vi "ToggleOnPress.vi"(11 "Input":bool) -> (3 "Output":bool)   [LabVIEW 2016]
doc: "Output becomes true Time Limit ms after Input becomes true and stays true"
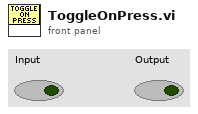
[diagram p1: front panel]
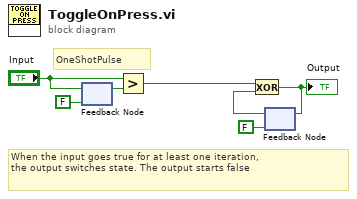
[diagram p0: block diagram]
diagram:
  # "OneShotPulse"
  # "When the input goes true for at least one iteration,\nthe output switches state. The output starts false"
  n1 = feedback-in #1("Input") -> ()
  n2 = feedback #1(FALSE ("Input")) -> (w7:bool)
  n3 = Greater?(x="Input", y=w7) -> (0:w1:bool)
  n4 = feedback #2(FALSE) -> (w2:bool)
  n5 = Exclusive Or(1:w2, 2:w1) -> (0:w3:bool)
  "Output" <- w3
  n6 = feedback-in #2(w3) -> ()
